vi "Parse Time String Array.vi"(4 "time":string[](array[string])) -> (1 "X-Axis Time":timestamp[](array[timestamp]))   [LabVIEW 2025, in "Weather Actor.lvlib" / "Weather.lvclass"]
uses:
  Weather.lvclass
  Weather.lvclass/Weather.ctl
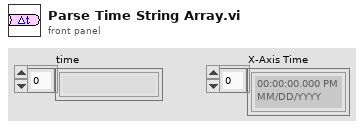
[diagram p1: front panel]
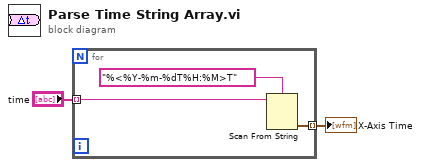
[diagram p0: block diagram]
diagram:
  n1 = for {
    tunnel: "time" -> [w4] mode=indexing
    tunnel: [w3] -> w1 mode=indexing
    n2 = Scan From String(format string="%<%Y-%m-%dT%H:%M>T", input string=w4) -> (output 1=w3:timestamp)  [unwired: 3 in, 3 out]
  }
  "X-Axis Time" <- w1
